vi "Get ID.vi"(8 "error in (no error)":errorcluster, 11 "hdl in":i32) -> (0 "error out":errorcluster, 2 "ID":string, 3 "hdl out":i32)   [LabVIEW 2011, in "Thorlabs_MDT69xB.lvlib"]
doc: "get the serial number of device."
uses:
  <instrlib>/Thorlabs_MDT69xB/Thorlabs_MDT69xB.lvlib
  <instrlib>/Thorlabs_MDT69xB/Data/MDT_COMMAND_LIB_win32.dll
  <instrlib>/Thorlabs_MDT69xB/Data/MDT_COMMAND_LIB_x64.dll
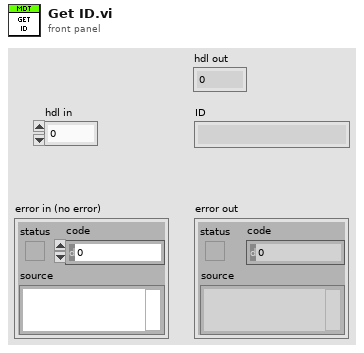
[diagram p1: front panel]
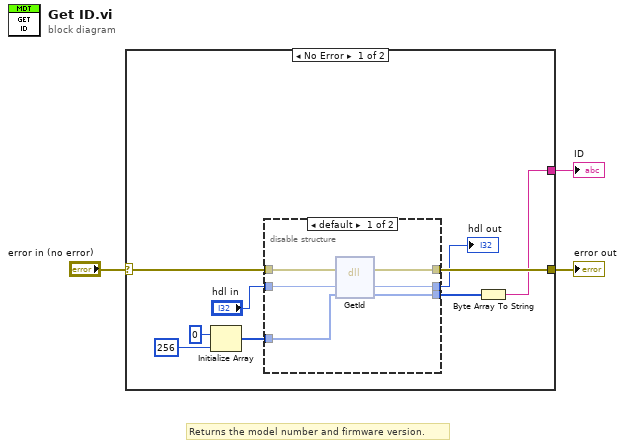
[diagram p0: block diagram]
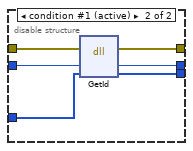
[diagram p2: hidden frame]
diagram:
  # "Returns the model number and firmware version."
  n1 = case shown="No Error" "error in (no error)" {
    selector: "error in (no error)" -> [w12 w25]
    tunnel: [w5 _] -> w3
    tunnel: [w11 w25] -> w2
    frame No Error {
      n2 = Initialize Array(u8 0 ("element"), 256 ("dimension size")) -> (w7:u8[])
      n3 = disable-structure shown="default" {
        disable-tunnel: w12 -> [w18 w24]
        disable-tunnel: [w17 w23] -> w11
        disable-tunnel: "hdl in" -> [w16 w22]
        disable-tunnel: w7 -> [w15 w21]
        disable-tunnel: [w14 w20] -> w6
        disable-tunnel: [w13 w19] -> w4
        frame condition #0 {
          n4 = dll-call lib="C:/Program Files (x86)/National Instruments/LabVIEW 2011/instr.lib/Thorlabs_MDT69xB/Data/MDT_COMMAND_LIB_win32.dll" fn="GetId"(error in=w18, "hdl"=w16, "id"=w15) -> (error out=w17:errorcluster, "hdl"=w13:i32, "id"=w14:u8[])  [unwired: 3 in, 1 out]
        }
        frame condition #1 (active) {
          n5 = dll-call lib="C:/Program Files/National Instruments/LabVIEW 2011/instr.lib/Thorlabs_MDT69xB/Data/MDT_COMMAND_LIB_x64.dll" fn="GetId"(error in=w24, "hdl"=w22, "id"=w21) -> (error out=w23:errorcluster, "hdl"=w19:i32, "id"=w20:u8[])  [unwired: 3 in, 1 out]
        }
      }
      "hdl out" <- w4
      n6 = Byte Array To String(unsigned byte array=w6) -> (string=w5:string)
    }
    frame Error {
    }
  }
  "ID" <- w3
  "error out" <- w2
